vi "Int2FXP_4ptMovAvg_Quantize.vi"(8 "Output Bit resolution":i8=12, 9 "Input Bit resolution":i8=12, 10 "Multiplier":fxp<+,8,4>=10.0 format="%#_19g", 11 "Input (Int)":i16) -> (3 "Output (FXP)":fxp<+/-,25,5>)   [LabVIEW 2019, in "FPGA functions.lvlib"]
doc: "Take a 4-point moving average and convert integer into Fixed Point (±16,5) \n\nSelect the appropriate quantization level."
uses:
  FPGA functions.lvlib
  <vilib>/Platform/TimedLoop/XDataNode/timing_clust.ctl
  <vilib>/Platform/TimedLoop/XDataNode/nitl_modes.ctl
  <vilib>/Platform/TimedLoop/XDataNode/wakeup.ctl
  <vilib>/rvi/Emulation/niFpgaSctlEmulationGetInTimedLoop.vi
  <vilib>/rvi/Emulation/niFpgaEmulationReportErrorSimple.vi
  <vilib>/rvi/Emulation/niFpgaGetClockAttributes.vi
  <vilib>/rvi/Emulation/niFpgaCriticalErrorInLSC.vi
  <vilib>/Platform/TimedLoop/XDataNode/XDataNode.xnode
  <vilib>/rvi/FXPMathLib/basic elements/FxpDiscreteDelay/XNode/nifxpmath_DiscreteDelay.xnode
  <vilib>/rvi/FXPMathLib/FxpMul/XNode/nifxpmath_Multiplier.xnode
  <vilib>/Platform/TimedLoop/XDataNode/XDNodeRunTimeDep.lvlib
  <vilib>/rvi/FXPMathLib/sim/FxpSim.dll
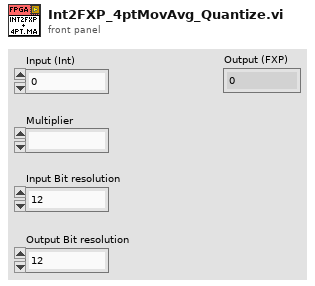
[diagram p1: front panel]
types:
  T1 = typedef "XDNodeRunTimeDep.lvlib/timing_clust.ctl" = cluster{"Expected End [f-1]":u64, "Actual End [f-1]":u64, "Finished Late? [f-1]":bool, "Expected End [i-1]":u64, "Actual End [i-1]":u64, "Finished Late? [i-1]":bool, "Expected Start [i]":u64, "Actual Start [i]":u64, "Expected Start [f]":u64, "Actual Start [f]":u64, "Source Name":string, "Structure Name":string, "Period":i64, "Deadline":i64, "Offset":i64, "Start":i64, "Priority":i32, "Timeout":i32, "Mode":T2, "Wakeup Reason":T3, "Error":errorcluster, "Source Type":string, "Secondary Source Type":string, "Global End Time":u64, "Global Start Time":u64, "Frame Duration":u64, "Iteration Duration":u64, "Assigned CPU":i32, "I/O Scan Engine Mode":u32}
  T2 = typedef "XDNodeRunTimeDep.lvlib/nitl_modes.ctl" = enum32{"No Change", "Process missed periods, maintain original phase", "Discard missed periods, maintain original phase", "Process missed periods, ignore original phase", "Discard missed periods, ignore original phase"}
  T3 = typedef "XDNodeRunTimeDep.lvlib/wakeup.ctl" = enum32{"Normal", "Aborted", "Asynchronous wakeup", "Timing source error", "Timed loop error", "Timeout"}
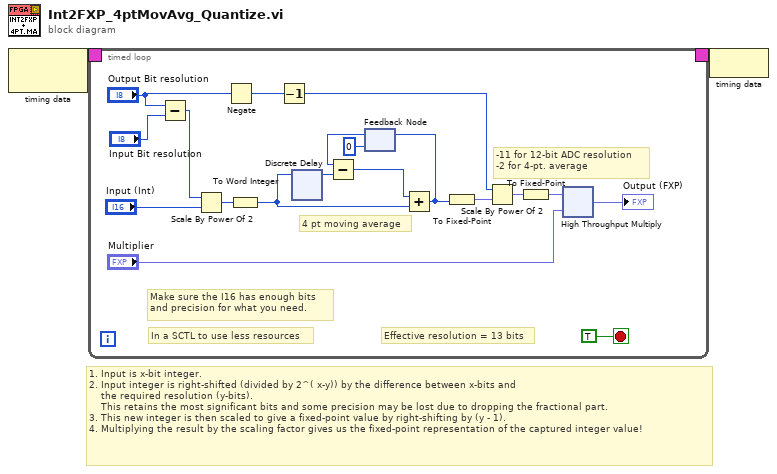
[diagram p0: block diagram]
diagram:
  # "1. Input is x-bit integer. \n2. Input integer is right-shifted (divided by 2^( x-y)) by the difference between x-bits and \n    the required resolution (y-bits).\n    This retains the most significant bits and some precision may be lost due to dropping the fractional part.\n3. This new integer is then scaled to give a fixed-point value by right-shifting by (y - 1).\n4. Multiplying the result by the scaling factor gives us the fixed-point representation of the captured integer value!"
  n1 = node-c288() -> (w2:T1)  [unwired: 1 in]
  n2 = timed-loop {
    timing: w2 -> [_]
    timing-out: [_] -> w1
    stop <- TRUE stop-if-true
    # "4 pt moving average"
    # "Effective resolution = 13 bits"
    # "-11 for 12-bit ADC resolution\n-2 for 4-pt. average"
    # "In a SCTL to use less resources"
    # "Make sure the I16 has enough bits \nand precision for what you need."
    n3 = Subtract(x="Output Bit resolution", y="Input Bit resolution") -> (x-y=w5:i8)
    n4 = Scale By Power Of 2(n=w5, x="Input (Int)") -> (x*2^n=w6:i16)
    n5 = Negate(x="Output Bit resolution") -> (-x=w3:i8)
    n6 = To Word Integer(number=w6) -> (16bit integer=w14:i16)
    n7 = Decrement(x=w3) -> (x-1=w4:i8)
    n8 = xnode ("Discrete Delay")("D"=w14) -> ("Q"=w17:i16)
    n9 = feedback #1(i16 0) -> (w15:i16)
    n10 = Subtract(x=w15, y=w17) -> (x-y=w16:i16)
    n11 = Add(x=w16, y=w14) -> (x+y=w12:i16)
    n12 = feedback-in #1(w12) -> ()
    n13 = To Fixed-Point(number=w12) -> (fixed-point=w8:fxp<+/-,32,16>)  [unwired: 1 in]
    n14 = Scale By Power Of 2(n=w4, x=w8) -> (x*2^n=w20:fxp<+/-,32,16>)
    n15 = To Fixed-Point(number=w20) -> (fixed-point=w19:fxp<+/-,18,1>)  [unwired: 1 in]
    n16 = xnode ("High Throughput Multiply")("x"=w19, "y"="Multiplier") -> ("x*y"=→"Output (FXP)":fxp<+/-,25,5>)
  }
  n17 = node-c288(w1) -> ()
